vi "Create Custom Sentry Array.vi"(11 "Custom Sentry Keys":string) -> (3 "Custom Sentry Key Array":string[](array[string]))   [LabVIEW 2025]
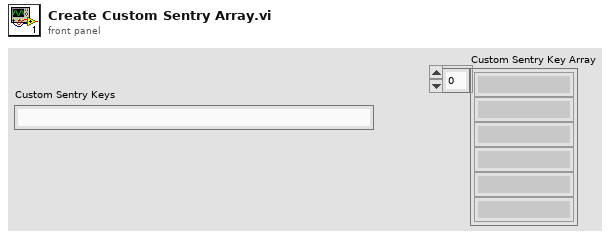
[diagram p1: front panel]
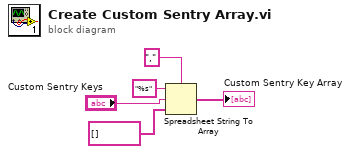
[diagram p0: block diagram]
diagram:
  n1 = Spreadsheet String To Array(delimiter (Tab)=",", format string="%s", spreadsheet string="Custom Sentry Keys", array type (2D Dbl)=string[] [] ("Array")) -> (array=→"Custom Sentry Key Array":string[])
